vi "Ejer4_tabla_Excel.vi"   [LabVIEW 2020]
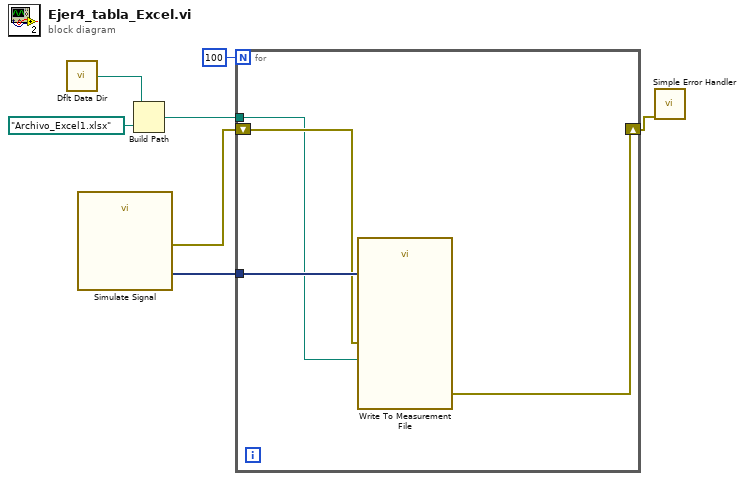
[diagram p0: block diagram]
diagram:
  n1 = call <vilib>:"Dflt Data Dir.vi"() -> ("App:Default Data Directory"=w3:path)
  n2 = call "Simulate Signal"() -> ("Sine"=w7:dynamicdata, "error out"=w5:errorcluster)  [unwired: 14 in]
  n3 = Build Path(base path=w3, name or relative path=path "Archivo_Excel1.xlsx") -> (appended path=w2:path)
  n4 = for {
    N: 100 -> [_]
    tunnel: w7 -> [w11]
    shift-right: [w9] -> w1
    shift-left: w5 -> [w10]
    tunnel: w2 -> [w8]
    n5 = call "Write To Measurement File"("Signals"=w11, "error in (no error)"=w10, "Filename"=w8) -> ("error out"=w9:errorcluster)  [unwired: 14 in, 2 out]
  }
  n6 = call <vilib>:"Simple Error Handler.vi"("error in (no error)"=w1) -> ()  [unwired: 4 in, 5 out]
